vi "To Variant.vi"(0 "Obj in":refnum<class "FSM.Node.lvclass">, 11 "error in (no error)":errorcluster) -> (4 "Obj out":refnum<class "FSM.Node.lvclass">, 8 "Array":variant[](array[variant]), 15 "error out":errorcluster)   [LabVIEW 2020, in "FSM.Node.lvclass"]
uses:
  FSM.Node.lvclass
  FSM.Node.lvclass/FSM.Node.ctl
  epl-vi-lib/Koop/KObject Class/KObject.lvclass
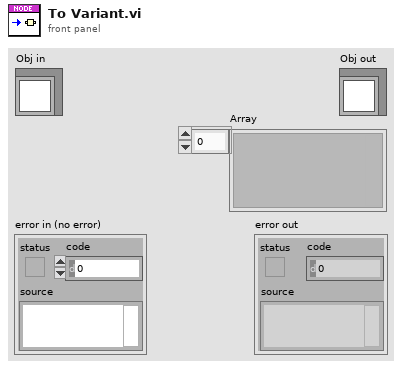
[diagram p1: front panel]
types:
  T1 = typedef "FSM.Node.lvclass/Serialized.ctl" = cluster{"Name":string, "BannerColor":u32, "Width":dbl, "Height":dbl, "FontSize":dbl, "Center":cluster{"X":dbl, "Y":dbl}, "Shape":T2, "Badges":T3[]}
  T2 = typedef "FSM.Node.lvclass/Shape.ctl" = enum16{"Default", "Start", "Action", "End"}
  T3 = typedef "FSM.Node.lvclass/Badge.ctl" = enum16{"Audio", "Visual"}
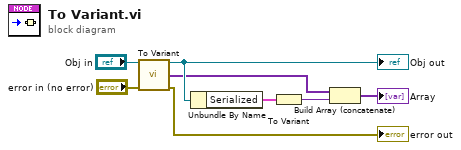
[diagram p0: block diagram]
diagram:
  n1 = call-parent "To Variant.vi"("KObject in"="Obj in", "error in (no error)"="error in (no error)") -> ("KObject out"=w3:refnum<class "FSM.Node.lvclass">, "Array"=w2:variant[], "error out"=→"error out":errorcluster)  [unwired: 11 in]
  "Obj out" <- w3
  n2 = Unbundle By Name(w3) -> ("Serialized"=w4:T1)
  n3 = To Variant(anything=w4) -> (Variant=w5:variant)
  n4 = Build Array (concatenate)(w2, w5) -> (→"Array":variant[])
